vi "Page_Advanced_WriteShared.vi"(6 "ctl references":T1, 8 "error in (no error)":errorcluster, 11 "AB_Application in":refnum<class "AB_Application.lvclass">) -> (0 "error out":errorcluster, 3 "AB_Application out":refnum<class "AB_Application.lvclass">)   [LabVIEW 2020, in "AB_Application.lvclass"]
uses:
  <vilib>/AppBuilder/AB_Classes/Application/AB_Application.lvclass
  <vilib>/AppBuilder/AB_Classes/Application/AB_Application.lvclass/AB_Application.ctl
  <resource>/Framework/Providers/Builds/AppBuilder/AB_UI_Page_Advanced_References.ctl
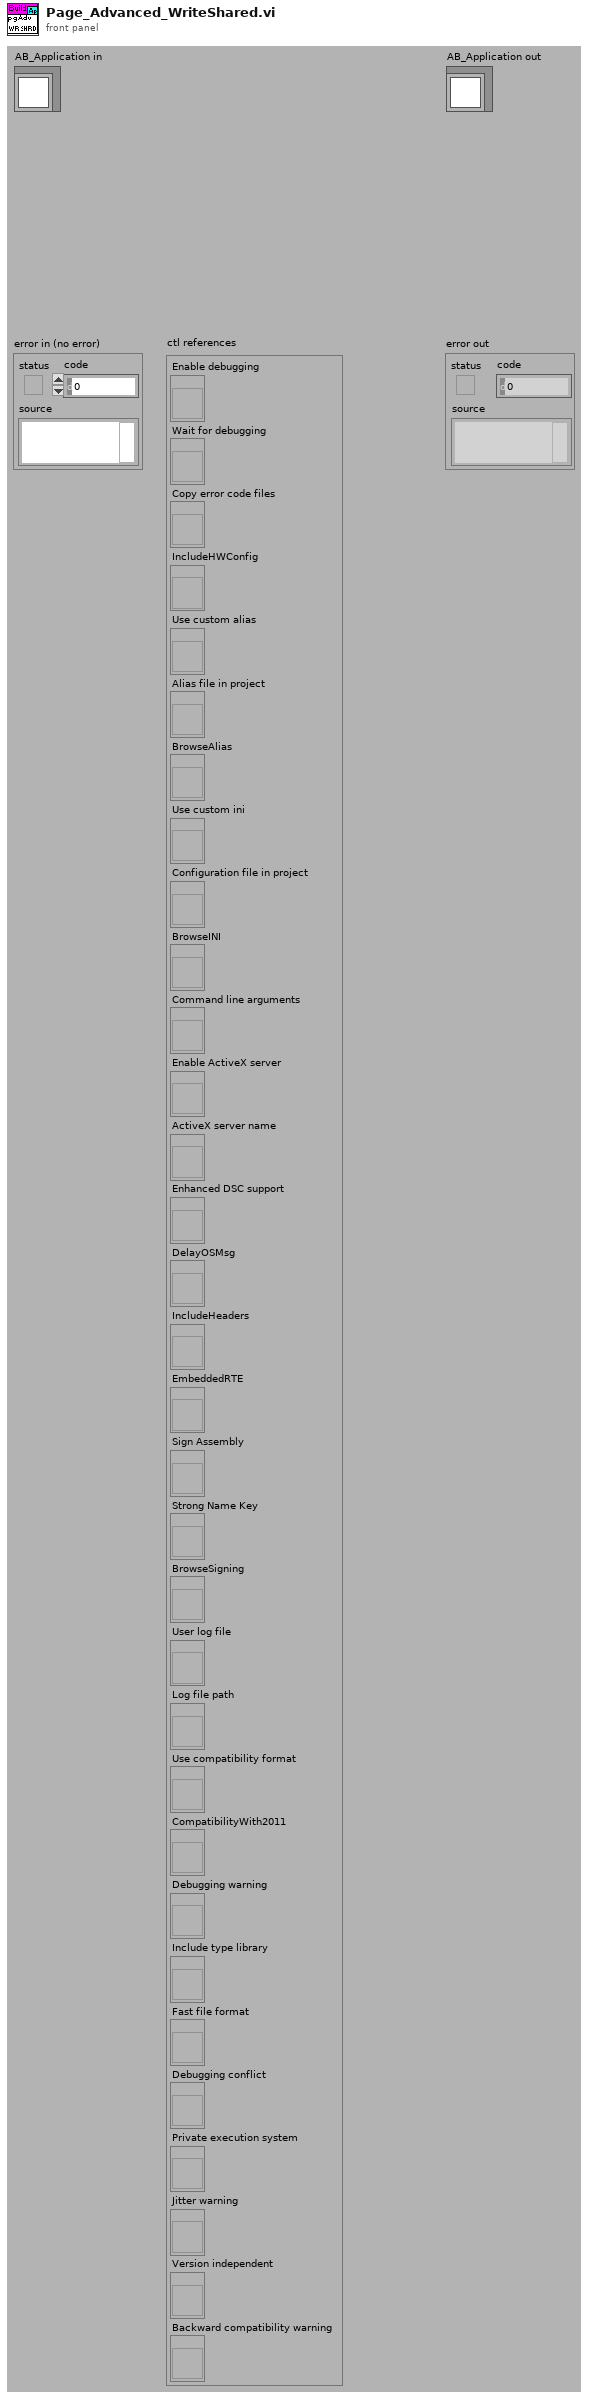
[diagram p1: front panel]
types:
  T1 = typedef "AB_UI_Page_Advanced_References.ctl" = cluster{"Enable debugging":refnum<vi>, "Wait for debugging":refnum<vi>, "Copy error code files":refnum<vi>, "IncludeHWConfig":refnum<vi>, "Use custom alias":refnum<vi>, "Alias file in project":refnum<vi>, "BrowseAlias":refnum<vi>, "Use custom ini":refnum<vi>, "Configuration file in project":refnum<vi>, "BrowseINI":refnum<vi>, "Command line arguments":refnum<vi>, "Enable ActiveX server":refnum<vi>, "ActiveX server name":refnum<vi>, "Enhanced DSC support":refnum<vi>, "DelayOSMsg":refnum<vi>, "IncludeHeaders":refnum<vi>, "EmbeddedRTE":refnum<vi>, "Sign Assembly":refnum<vi>, "Strong Name Key":refnum<vi>, "BrowseSigning":refnum<vi>, "User log file":refnum<vi>, "Log file path":refnum<vi>, "Use compatibility format":refnum<vi>, "CompatibilityWith2011":refnum<vi>, "Debugging warning":refnum<vi>, "Include type library":refnum<vi>, "Fast file format":refnum<vi>, "Debugging conflict":refnum<vi>, "Private execution system":refnum<vi>, "Jitter warning":refnum<vi>, "Version independent":refnum<vi>, "Backward compatibility warning":refnum<vi>}
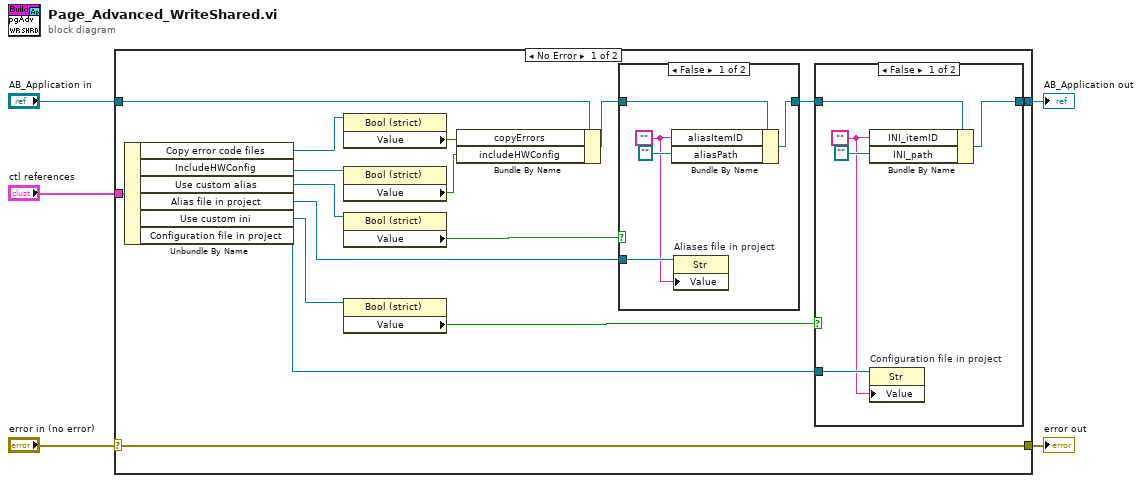
[diagram p0: block diagram]
diagram:
  n1 = case shown="No Error" "error in (no error)" {
    selector: "error in (no error)" -> [w21 w35]
    tunnel: [w21 w35] -> w4
    tunnel: [w8 w34] -> w2
    tunnel: "AB_Application in" -> [w20 w34]
    tunnel: "ctl references" -> [w19 _]
    frame No Error {
      n2 = Unbundle By Name(w19) -> ("Copy error code files"=w18:refnum<vi>, "IncludeHWConfig"=w16:refnum<vi>, "Use custom alias"=w14:refnum<vi>, "Alias file in project"=w10:refnum<vi>, "Use custom ini"=w11:refnum<vi>, "Configuration file in project"=w6:refnum<vi>)
      n3 = property class="Bool (strict)"(reference=w18) -> ("Value"=w17:bool)  [unwired: 1 in, 2 out]
      n4 = property class="Bool (strict)"(reference=w16) -> ("Value"=w15:bool)  [unwired: 1 in, 2 out]
      n5 = property class="Bool (strict)"(reference=w14) -> ("Value"=w12:bool)  [unwired: 1 in, 2 out]
      n6 = property class="Bool (strict)"(reference=w11) -> ("Value"=w7:bool)  [unwired: 1 in, 2 out]
      n7 = Bundle By Name(cluster=w20, "copyErrors"=w17, "includeHWConfig"=w15) -> (w13:refnum<class "AB_Application.lvclass">)
      n8 = case shown="False" w12 {
        tunnel: w13 -> [w32 w33]
        tunnel: [w31 w33] -> w9
        tunnel: w10 -> [w29 _]
        frame False {
          w28 = ""
          n9 = Bundle By Name(cluster=w32, "aliasItemID"=w28, "aliasPath"=path "") -> (w31:refnum<class "AB_Application.lvclass">)
          n10 = property on="Aliases file in project" class="Str"(reference=w29, "Value"=w28) -> ()  [unwired: 1 in, 2 out]
        }
        frame True {
        }
      }
      n11 = case shown="False" w7 {
        tunnel: w9 -> [w26 w27]
        tunnel: [w25 w27] -> w8
        tunnel: w6 -> [w23 _]
        frame False {
          w22 = ""
          n12 = Bundle By Name(cluster=w26, "INI_itemID"=w22, "INI_path"=path "") -> (w25:refnum<class "AB_Application.lvclass">)
          n13 = property on="Configuration file in project" class="Str"(reference=w23, "Value"=w22) -> ()  [unwired: 1 in, 2 out]
        }
        frame True {
        }
      }
    }
    frame Error {
    }
  }
  "error out" <- w4
  "AB_Application out" <- w2
